vi "Set Gear Ratio.vi"(6 "subpanel to main command event":T1, 8 "error in (no error)":errorcluster, 10 "gear ratio":dbl, 11 "steering frame ref in":refnum<data-value>) -> (0 "error out":errorcluster, 3 "steering frame ref out":refnum<data-value>)   [LabVIEW 2017, in "NI_Robotics_Configure Steering Frame.lvlib" / "Differential Frame Subpanel.lvlib"]
uses:
  <vilib>/robotics/Dialog/Configure Steering Frame/Differential Frame Subpanel/Differential Frame Subpanel.lvlib
  <vilib>/robotics/Steering/Differential Steering Frame/NI_Robotics_Differential Steering Frame.lvclass
  c:/Program Files (x86)/National Instruments/LabVIEW 2017/vi.lib/robotics/Steering/Steering Frame/NI_Robotics_Steering Frame.lvclass
  <vilib>/robotics/Dialog/Configure Steering Frame/Subpanel to Main Command Event.ctl
  <vilib>/robotics/Dialog/Configure Steering Frame/Subpanel to Main Command.ctl
  <vilib>/robotics/Dialog/Configure Steering Frame/Generate Subpanel to Main Event.vi
  <vilib>/robotics/Steering/Steering Frame/NI_Robotics_Steering Frame.lvclass
  <vilib>/robotics/Dialog/Configure Steering Frame/NI_Robotics_Configure Steering Frame.lvlib
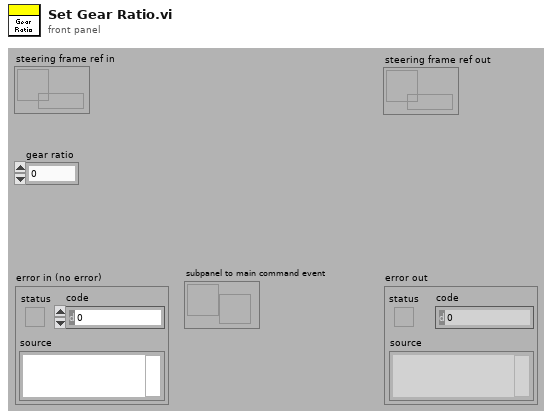
[diagram p1: front panel]
types:
  T1 = typedef "NI_Robotics_Configure Steering Frame.lvlib/Subpanel to Main Command Event.ctl" = refnum<user-event>
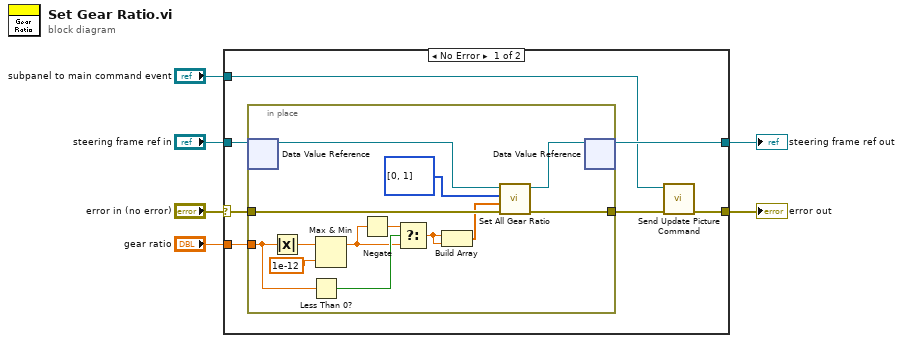
[diagram p0: block diagram]
diagram:
  n1 = case shown="No Error" "error in (no error)" {
    selector: "error in (no error)" -> [w11 w27]
    tunnel: "steering frame ref in" -> [w13 w28]
    tunnel: [w12 w28] -> w4
    tunnel: [w7 w27] -> w3
    tunnel: "gear ratio" -> [w10 _]
    tunnel: "subpanel to main command event" -> [w9 _]
    frame No Error {
      n2 = in-place {
        in-place-border: w11 -> [w25]
        in-place-border: w10 -> [w18]
        in-place-border: [w22] -> w8
        n3 = in-place-dvr #1(w13) -> (w26:refnum<class "NI_Robotics_Differential Steering Frame.lvclass">)  [unwired: 1 out]
        n4 = Absolute Value(x=w18) -> (abs(x)=w20:dbl)
        n5 = Less Than 0?(x=w18) -> (x < 0?=w17:bool)
        n6 = Max & Min(x=w20, y=1e-12) -> (max(x,y)=w15:dbl)  [unwired: 1 out]
        n7 = Negate(x=w15) -> (-x=w14:dbl)
        n8 = Select(t=w14, s=w17, f=w15) -> (s? t:f=w16:dbl)
        n9 = Build Array(w16, w16) -> (w21:dbl[])
        n10 = call <vilib>:"Set All Gear Ratio.vi"("error in (no error)"=w25, "gear ratio"=w21, "wheel indexes"=i32[] [0, 1], "steering frame in"=w26) -> ("error out"=w22:errorcluster, "steering frame out"=w23:refnum<class "NI_Robotics_Differential Steering Frame.lvclass">)  [unwired: 5 in, 1 out]
        n11 = in-place-dvr #1(w23) -> (w12:refnum<data-value>)  [unwired: 1 out]
      }
      n12 = call <vilib>:"Send Update Picture Command.vi"("error in (no error)"=w8, "subpanel to main command event"=w9) -> ("error out"=w7:errorcluster)  [unwired: 9 in]
    }
    frame Error {
    }
  }
  "steering frame ref out" <- w4
  "error out" <- w3
